vi "create_displayable_msg.vi"(9 "pad_with_spaces (T)":bool=TRUE, 10 "separator (none)":T1(ring), 11 "Error in":refnum<class "Error.lvclass">) -> (3 "error_msg_to_display":string)   [LabVIEW 2023, in "Error Handling Interface.lvlib" / "Error.lvclass"]
doc: "From the object, builds a decoded, <B>user-friendly</B> message"
uses:
  Error.lvclass
  Error.lvclass/Error.ctl
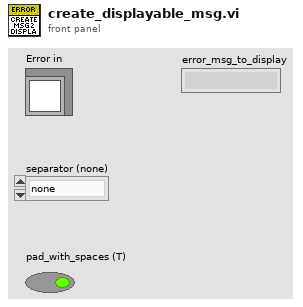
[diagram p1: front panel]
types:
  T1 = enum16{"none", "hifen", "fslash", "bslash", "vbar", "dot", "comma"}
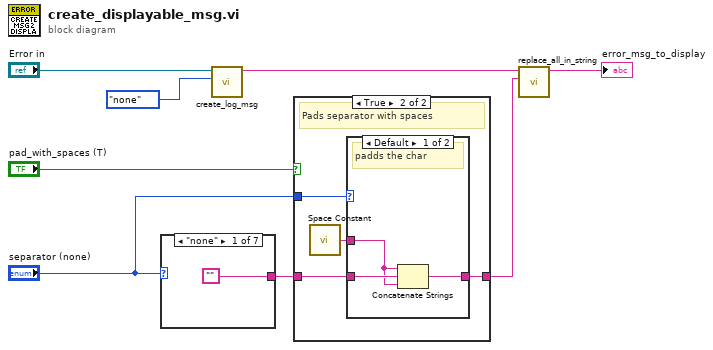
[diagram p0: block diagram]
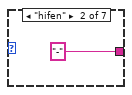
[diagram p4: hidden frame]
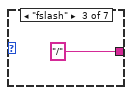
[diagram p5: hidden frame]
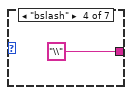
[diagram p6: hidden frame]
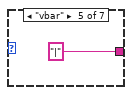
[diagram p7: hidden frame]
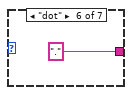
[diagram p8: hidden frame]
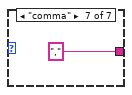
[diagram p9: hidden frame]
diagram:
  n1 = case shown="\"none\"" "separator (none)" {
    tunnel: ["" "-" "/" "\\" "|" "." ","] -> w6
    frame "none" {
    }
    frame "hifen" {
    }
    frame "fslash" {
    }
    frame "bslash" {
    }
    frame "vbar" {
    }
    frame "dot" {
    }
    frame "comma" {
    }
  }
  n2 = call "create_log_msg.vi"("string_type"=enum16{"none", "csv", "json", "xml"}."none" ("string_type (csv)"), "Error in"="Error in") -> ("error_msg_to_log"=w1:string)  [unwired: 9 in]
  n3 = case shown="True" "pad_with_spaces (T)" {
    tunnel: [w16 w19] -> w7
    tunnel: w6 -> [w16 w20]
    tunnel: "separator (none)" -> [_ w17]
    frame False {
      # "forwards separator as selected"
    }
    frame True {
      # "Pads separator with spaces"
      n4 = call <vilib>:"Space Constant.vi"() -> ("String"=w18:string)
      n5 = case shown="Default" w17 {
        tunnel: w20 -> [w23 _]
        tunnel: [w22 w24] -> w19
        tunnel: w18 -> [w21 w24]
        frame Default {
          # "padds the char"
          n6 = Concatenate Strings(w21, w23, w21) -> (w22:string)
        }
        frame "none" {
          # "adds only a single space"
        }
      }
    }
  }
  n7 = call "replace_all_in_string.vi"("replace_string"=w7, "string_in"=w1) -> ("string_out"=→"error_msg_to_display":string)  [unwired: 9 in]
